vi "Wind2Wrap.vi"(4 "In":dbl) -> (1 "Out":dbl)   [LabVIEW 2015]
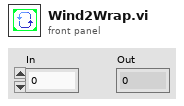
[diagram p1: front panel]
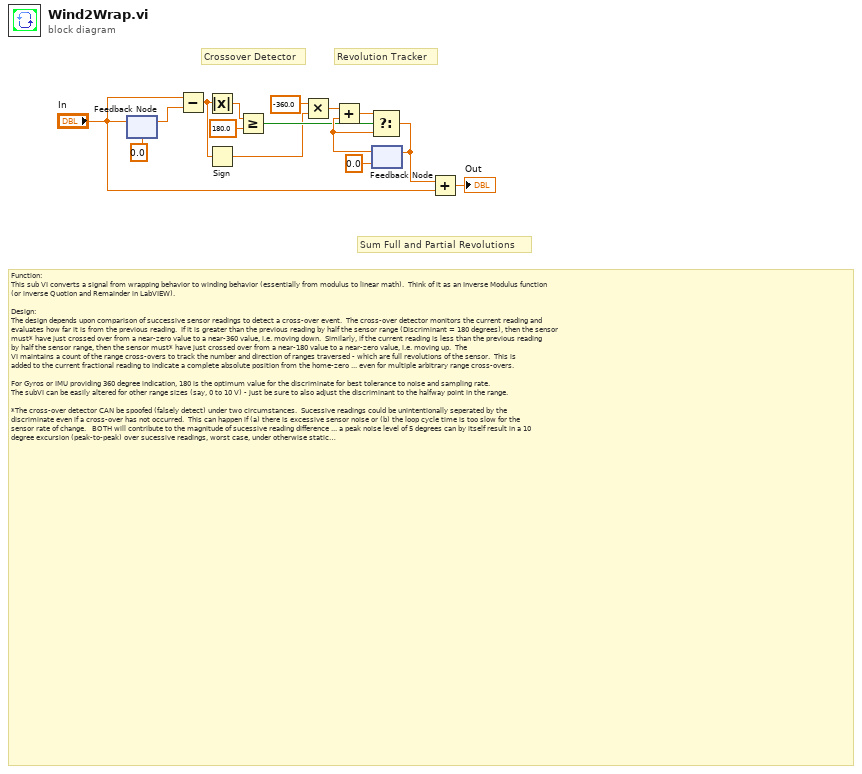
[diagram p0: block diagram]
diagram:
  # "Sum Full and Partial Revolutions"
  # "Revolution Tracker"
  # "Crossover Detector"
  # "Function:\nThis sub VI converts a signal from wrapping behavior to winding behavior (essentially from modulus to linear math).  Think of it as an Inverse Modulus function\n(or inverse Quotion and Remainder in LabVIEW).\n\nDesign:\nThe design depends upon comparison of successive sensor readings to detect a cross-over event.  The cross-over detector monitors the current reading and \nevaluates how far it is from the previous reading.  If it is greater than the previous reading by half the sensor range (Discriminant = 180 degrees), then the sensor \nmust* have just crossed over from a near-zero value to a near-360 value, i.e. moving down.  Similarly, if the current reading is less than the previous reading\nby half the sensor range, then the sensor must* have just crossed over from a near-180 value to a near-zero value, i.e. moving up.  The \nVI maintains a count of the range cross-overs to track the number and direction of ranges traversed - which are full revolutions of the sensor.  This is \nadded to the current fractional reading to indicate a complete absolute position from the home-zero ... even for multiple arbitrary range cross-overs.\n\nFor Gyros or IMU providing 360 degree indication, 180 is the optimum value for the discriminate for best tolerance to noise and sampling rate.\nThe subVI can be easily altered for other range sizes (say, 0 to 10 V) - just be sure to also adjust the discriminant to the halfway point in the range. \n\n*The cross-over detector CAN be spoofed (falsely detect) under two circumstances.  Sucessive readings could be unintentionally seperated by the\ndiscriminate even if a cross-over has not occurred.  This can happen if (a) there is excessive sensor noise or (b) the loop cycle time is too slow for the \nsensor rate of change.   BOTH will contribute to the magnitude of sucessive reading difference ... a peak noise level of 5 degrees can by itself result in a 10 \ndegree excursion (peak-to-peak) over sucessive readings, worst case, under otherwise static conditions.  The cycle time for the loop where the sensor read is \nlocated effectively limits the sampling rate while the sensor value is changing - slow sampling of a relatively fast moving reading can also produce a large \ndifference in sucessive readings, which can fool the cross-over detector into missing cross-over events.\n\nTo prevent the possibility of these cross-over false detects, the sampling rate / loop cycle time must be sufficiently fast given the amount of peak noise \npresent and the maximum rate at which the sensor might rotate.   The principle is that the peak-to-peak noise plus the product of the max sensor rate of \nchange and the loop period must be less than the discriminant.  Solving for the loop period ...\n\n                                                           Loop Period < (180 - 2*n) / (360 * Sensor RPS)\nwhere:\n                                                           n = peak noise level, in degrees\n                                                           Sensor RPS = maximum rate the sensor might change, in revolutions per second\n                                                           Loop Period = minimum required sampling rate of sensor, in seconds\n\nTeam 836 The RoboBees ...  Orient your behavior to move beyond your current confines, grow into a STEM field!"
  n1 = feedback #1(0.0) -> (w13:dbl)
  n2 = feedback-in #1("In") -> ()
  n3 = Subtract(x="In", y=w13) -> (x-y=w3:dbl)
  n4 = Absolute Value(x=w3) -> (abs(x)=w9:dbl)
  n5 = Sign(1:w3) -> (0:w2:dbl)
  n6 = Greater Or Equal?(x=w9, y=180.0) -> (x >= y?=w4:bool)
  n7 = Multiply(x=-360.0 ("y"), y=w2) -> (x*y=w11:dbl)
  n8 = feedback #2(0.0) -> (w8:dbl)
  n9 = Add(x=w11, y=w8) -> (x+y=w12:dbl)
  n10 = Select(t=w12, s=w4, f=w8) -> (s? t:f=w5:dbl)
  n11 = feedback-in #2(w5) -> ()
  n12 = Add(x=w5, y="In") -> (x+y=→"Out":dbl)
